vi "offset_lat-long.vi"(1 "gps offset":dbl, 2 "lat/lon position":T1) -> (0 "Cluster":T1)   [LabVIEW 2020]
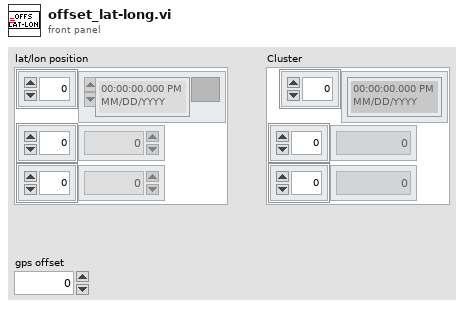
[diagram p1: front panel]
types:
  T1 = cluster{"Array":timestamp[], "Array":dbl[], "Array":dbl[]}
  T2 = cluster{timestamp[], "Array":dbl[], "Array":dbl[]}
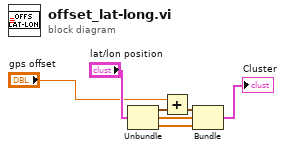
[diagram p0: block diagram]
diagram:
  n1 = Unbundle("lat/lon position") -> ("Array"=w1:timestamp[], "Array"=w5:dbl[], "Array"=w6:dbl[])
  n2 = Add(x="gps offset", y=w1) -> (x+y=w3:timestamp[])
  n3 = Bundle(w3, "Array"=w5, "Array"=w6) -> (→"Cluster":T2)  [unwired: 1 in]
